vi "Ball Intake Routine.vi"   [LabVIEW 2018]
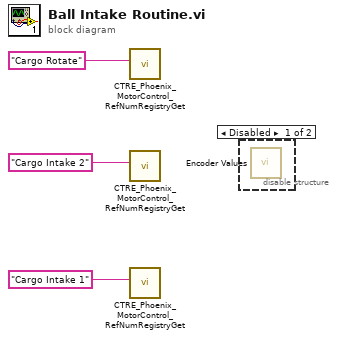
[diagram p0: block diagram]
diagram:
  n1 = call <vilib>:"CTRE_Phoenix_MotorControl_RefNumRegistryGet.vi"("refnum name"="Cargo Rotate") -> ()  [unwired: 9 in, 2 out]
  n2 = call <vilib>:"CTRE_Phoenix_MotorControl_RefNumRegistryGet.vi"("refnum name"="Cargo Intake 2") -> ()  [unwired: 9 in, 2 out]
  n3 = call <vilib>:"CTRE_Phoenix_MotorControl_RefNumRegistryGet.vi"("refnum name"="Cargo Intake 1") -> ()  [unwired: 9 in, 2 out]
  n4 = disable-structure shown="Disabled" {
    frame Disabled {
      n5 = call "Encoder Values.vi"() -> ()  [unwired: 9 in, 3 out]
    }
    frame Enabled {
    }
  }
